vi "Intake_Ball_Set.vi"() -> ()   [LabVIEW 2018]
uses:
  Intake_Ball_Control_Type.ctl
  <vilib>/Rock Robotics/WPI/DriverStation/WPI_DriverStationRobotMode2.ctl
  Global_Variables/Intake_Ball_Globals.vi
  Global_Variables/Robot_Global_Data.vi
  Global_Variables/Sensor_Values.vi
  Global_Variables/Autonomous_Globals.vi
panel:
  in  "Threshold":dbl=1.0
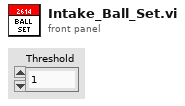
[diagram p1: front panel]
types:
  T1 = typedef "Intake_Ball_Control_Type.ctl" = enum16{"No_Op", "Manual_In", "Manual_Out", "In_Sensor_Stop", "Out_Teleop", "Out", "Stall"}
  T2 = typedef "WPI_DriverStationRobotMode2.ctl" = enum16{"Autonomous Disabled", "Autonomous Enabled", "Teleop Disabled", "Teleop Enabled", "Disconnected", "Finish", "Test Disabled", "Test Enabled", "Emergency Stopped"}
  T3 = typedef "Intake_Ball_Notifier.ctl" = cluster{"Intake_Ball_Control_Type":T1, "Manual_In":bool, "Manual_Out":bool, "Ball_In":bool, "Ball_Out":bool, "Parameter_One":dbl, "Parameter_Two":dbl, "Parameter_Three":dbl, "Step":i32, "Ball_Notifier":refnum<notifier>}
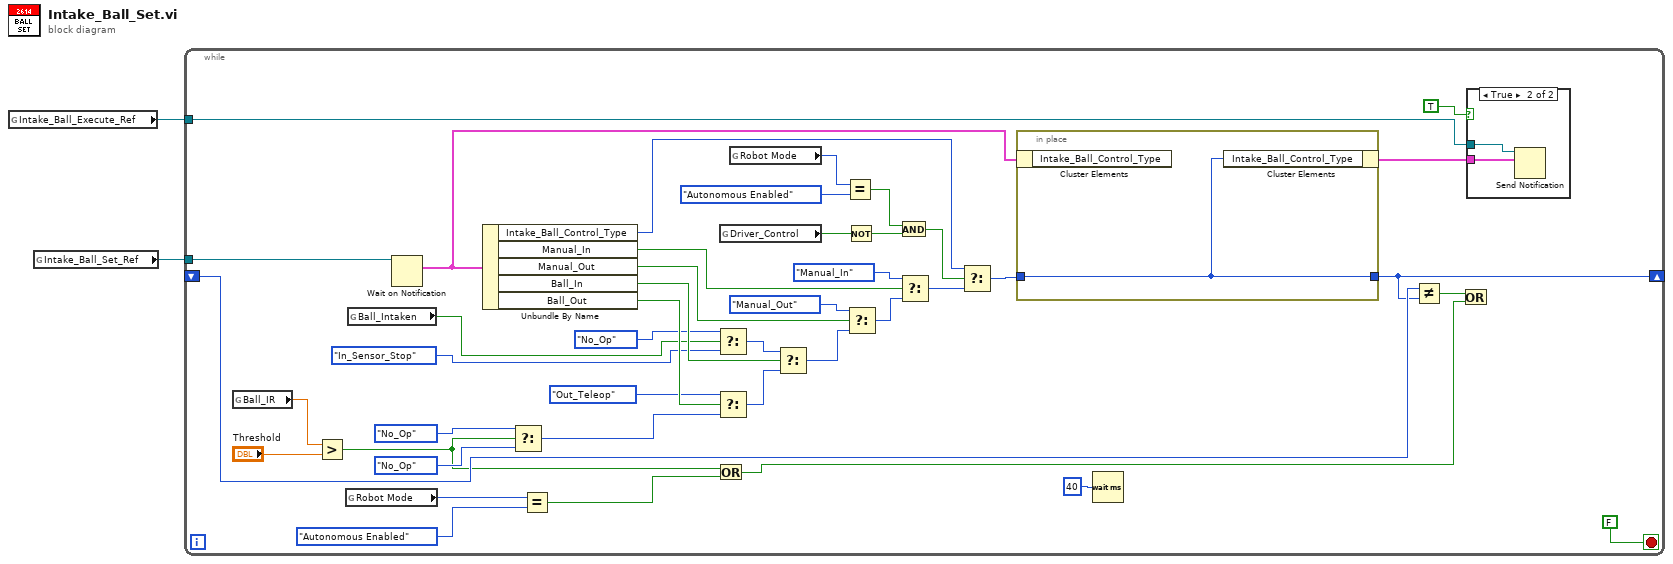
[diagram p0: block diagram]
diagram:
  n1 = global read "Intake_Ball_Globals.vi" "Intake_Ball_Execute_Ref"() -> (w1:refnum<notifier>)
  n2 = global read "Intake_Ball_Globals.vi" "Intake_Ball_Set_Ref"() -> (w2:refnum<notifier>)
  n3 = while {
    tunnel: w2 -> [w43]
    tunnel: w1 -> [w41]
    shift-right: [w23] -> _
    shift-left: _ -> [w24]
    stop <- FALSE stop-if-true
    n4 = global read "Sensor_Values.vi" "Ball_IR"() -> (w13:dbl)
    n5 = Greater?(x=w13, y="Threshold") -> (0:w9:bool)
    n6 = global read "Robot_Global_Data.vi" "Robot Mode"() -> (w20:T2)
    n7 = global read "Sensor_Values.vi" "Ball_Intaken"() -> (w18:bool)
    n8 = Wait on Notification(notifier=w43) -> (notification=w42:T3)  [unwired: 3 in, 3 out]
    n9 = Unbundle By Name(w42) -> ("Intake_Ball_Control_Type"=w37:T1, "Manual_In"=w34:bool, "Manual_Out"=w33:bool, "Ball_In"=w28:bool, "Ball_Out"=w26:bool)
    n10 = Select(t=Intake_Ball_Control_Type."No_Op", s=w9, f=Intake_Ball_Control_Type."No_Op" ("Intake_Ball_Control_Type")) -> (s? t:f=w11:T1)
    n11 = Equal?(x=w20, y=WPI_DriverStationRobotMode2."Autonomous Enabled") -> (x = y?=w19:bool)
    n12 = Or(x=w9, y=w19) -> (x .or. y?=w14:bool)
    n13 = Select(t=Intake_Ball_Control_Type."No_Op", s=w18, f=Intake_Ball_Control_Type."In_Sensor_Stop" ("Intake_Ball_Control_Type")) -> (s? t:f=w17:T1)
    n14 = Select(t=Intake_Ball_Control_Type."Out_Teleop", s=w26, f=w11) -> (s? t:f=w27:T1)
    n15 = global read "Autonomous_Globals.vi" "Driver_Control"() -> (w5:bool)
    n16 = global read "Robot_Global_Data.vi" "Robot Mode"() -> (w39:T2)
    n17 = Select(t=w17, s=w28, f=w27) -> (s? t:f=w29:T1)
    n18 = Equal?(x=w39, y=WPI_DriverStationRobotMode2."Autonomous Enabled") -> (x = y?=w4:bool)
    n19 = Not(x=w5) -> (.not. x?=w6:bool)
    n20 = Select(t=Intake_Ball_Control_Type."Manual_Out", s=w33, f=w29) -> (s? t:f=w32:T1)
    n21 = And(x=w4, y=w6) -> (x .and. y?=w3:bool)
    n22 = Select(t=Intake_Ball_Control_Type."Manual_In", s=w34, f=w32) -> (s? t:f=w35:T1)
    n23 = Select(t=w37, s=w3, f=w35) -> (s? t:f=w40:T1)
    n24 = in-place {
      in-place-border: w40 -> [w48]
      in-place-border: [w48] -> w23
      n25 = in-place-cluster #1(w42) -> ()  [unwired: 1 out]
      n26 = in-place-cluster #1("Intake_Ball_Control_Type"=w48) -> (w36:T3)
    }
    n27 = Wait (ms)(milliseconds to wait=u32 40) -> ()  [unwired: 1 out]
    n28 = Not Equal?(x=w24, y=w23) -> (x != y?=w22:bool)
    n29 = Or(x=w22, y=w14) -> ()  [unwired: 1 out]
    n30 = case shown="True" TRUE {
      tunnel: w41 -> [_ w47]
      tunnel: w36 -> [_ w46]
      frame False {
      }
      frame True {
        n31 = Send Notification(notification=w46, notifier=w47) -> ()  [unwired: 1 in, 2 out]
      }
    }
  }
